vi "Stimulus-Plot (full).vi"(0 "AO Control":T1[](xcontrol), 1 "Waveform Graph":refnum<vi>, 5 "Array":dbl[][](array[numeric]), 9 "Sampling Rate (Hz)":dbl, 11 "error in (no error)":errorcluster, 12 "Decorations[]":refnum<vi>[](array[refnum])) -> (4 "AO Control out":T1[](xcontrol), 6 "Array out":dbl[][](array[numeric]), 15 "error out":errorcluster)   [LabVIEW 2020]
doc: "Helper function to plot stimuli in a sensible fashion."
uses:
  Controls/Multichannel (Full)/Multichannel (Full).xctl
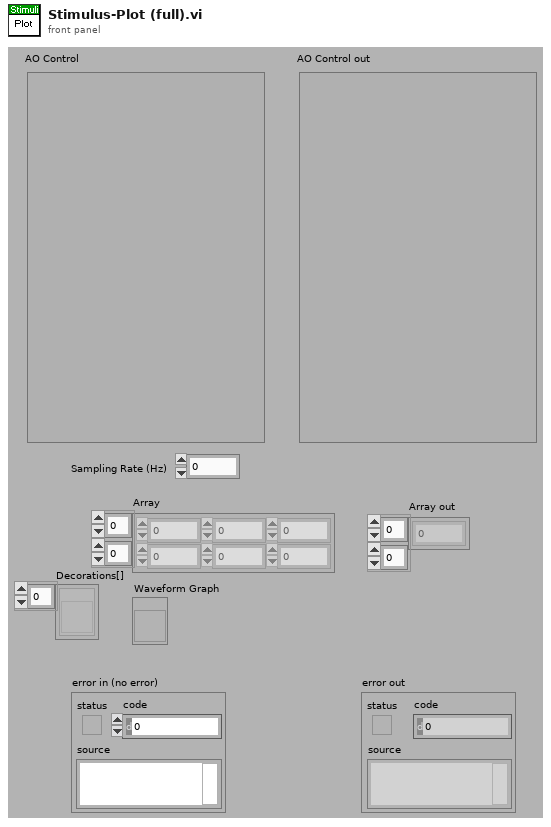
[diagram p1: front panel]
types:
  T1 = typedef "Stimulus Channel (Full).xctl/Full Stimulus Channel Data.ctl" = cluster{"Waveform":T2, "Filter":T19, "Burst":T21, "Level":T22, "Name":string, "Advanced":T24, "SAM":T25}
  T2 = typedef "Waveform XCtl.xctl/Waveform Data.ctl" = cluster{"Type":T3, "Tone":T4, "Pulse Train":T5, "Noise":T8, "File":T9, "FMSweep":T10, "Chirp Train":T11, "Complex Tone":cluster{"Params":T13, "Data":T15}, "Moving Ripple":T16}
  T3 = typedef "Waveform Enum.ctl" = enum16{"OFF", "Tone", "Noise", "Pulse Train", "File", "FM Sweep", "Chirp Train", "Complex Tone", "FM Tone", "Moving Ripple"}
  T4 = typedef "Tone Params.ctl" = cluster{"Frequency (kHz)":dbl, "Last Freq":dbl, "Last Phase":dbl}
  T5 = typedef "Pulse Train Params.ctl" = cluster{"Pulse width (us)":dbl, "Pulse rate (Hz)":dbl, "Gap (ms)":dbl, "Polarity":T6, "PT State":T7, "Asynch":bool}
  T6 = typedef "Pulse Polarity.ctl" = enum16{"POS", "NEG", "POS-NEG", "NEG-POS"}
  T7 = typedef "PT-Continuous State.ctl" = cluster{"Template":dbl[], "Nperiod":i32, "Index":i32, "Pulse Rate (Hz)":dbl, "Phase (cycles)":dbl, "Noff":i32}
  T8 = typedef "Noise Params.ctl" = cluster{"InvFilt":bool, "Noise":dbl[], "CurPt":i32, "Aweight":bool, "Seed":i32, "afile":path}
  T9 = typedef "StimFile-Params.ctl" = cluster{"Filename":path, "Signal":dbl[], "Channel":i32, "stream":bool, "offset":i32, "nreps":i32, "loops":i32, "Randomize":bool, "order":i32[], "Seed":i32, "Tokens":i32}
  T10 = typedef "FM Sweep Params.ctl" = cluster{"Rate (oct/s)":dbl, "Fmin (Hz)":dbl, "Fmax (Hz)":dbl, "Ramp (ms)":dbl, "Linear":bool}
  T11 = typedef "Chirp Train.ctl" = cluster{"Params":T12, "Data":cluster{"WF":dbl[]}}
  T12 = typedef "Chirp Train Params.ctl" = cluster{"Fmin (kHz)":dbl, "Fmax (kHz)":dbl, "Compensate":bool, "Duration (ms)":dbl}
  T13 = typedef "CT-Params.ctl" = cluster{"F0 (Hz)":dbl, "Band":cluster{"Flow (Hz)":dbl, "Fhigh (Hz)":dbl}, "Phase":T14, "Min F0 (Hz)":dbl, "Max F0 (Hz)":dbl, "ContinRandPhase":bool, "Max peak factor":dbl, "Max mod depth":dbl, "MinHarmNum":i32, "MaxHarmNum":i32, "Level Mode":enum16{"per component", "overall rms"}, "% jitter":dbl}
  T14 = typedef "CT-Phase Enum.ctl" = enum16{"Cosine", "Random", "Alternating"}
  T15 = typedef "CT-Runtime Data.ctl" = cluster{"Ncomp":i32, "MinHarm":i32, "Phase":dbl[], "Amplitude":dbl[], "Npts/frame":i32, "Last F0":dbl, "Fmin":dbl, "Fmax":dbl, "Lslope":dbl, "randphase":bool, "overall rms":bool, "fmult":dbl[], "jittered":bool}
  T16 = typedef "Moving Ripple.ctl" = cluster{"Params":T17, "Data":T18}
  T17 = typedef "Moving Ripple.Params.ctl" = cluster{"Fmin":dbl, "Fmax":dbl, "Density":dbl, "Velocity":dbl, "Depth":dbl, "Phase":dbl, "Comp/oct":i32}
  T18 = typedef "Moving Ripple.Data.ctl" = cluster{"Freq":dbl[], "A":dbl[], "phase":dbl[], "Phase":dbl}
  T19 = typedef "Advanced Filter XCtl.xctl/Filter Data.ctl" = cluster{"Type":enum16{"Lowpass", "Highpass", "Bandpass", "Bandstop", "OFF"}, "CF (kHz)":dbl, "BW (kHz)":dbl, "Cascade":bool, "Quadrature":bool, "Scale Factor":dbl, "Stages":cluster{"IIR Filter":cluster{"filter structure":enum32{"IIR 2nd Order", "IIR 4th Order"}, "Reverse Coefficients":dbl[], "Forward Coefficients":dbl[]}, "State":dbl[]}[], "Class":enum16{"Elliptic", "Butterworth"}, "Order":i32, "BWUnits":T20}
  T20 = typedef "Filter-Bandwidth Units.ctl" = enum16{"Linear", "Octaves", "Min-Max"}
  T21 = typedef "Burst Control.xctl/Burst Data.ctl" = cluster{"Active":bool, "Delay (ms)":dbl, "Duration (ms)":dbl, "Ramp (ms)":dbl, "Rate (Hz)":dbl, "Trepeat (ms)":dbl, "Repeat":bool}
  T22 = typedef "Level XCtl.xctl/Level Data.ctl" = cluster{"Level":dbl, "Units":T23, "Max":dbl, "Multiplier":dbl, "Cal File":path, "Cal":cluster{"Freq (Hz)":dbl[], "Mag (dB SPL)":dbl[], "Phase (deg)":dbl[]}}
  T23 = typedef "Level Units.ctl" = enum16{"dB atten", "dB SPL", "dB re 1 Vrms", "dB V/Hz½", "mW", "dB HL", "Volts", "dB mW"}
  T24 = typedef "Advanced Stimulus Options.xctl/Advanced Stimulus Options.ctl" = cluster{"Rep Mask":string, "AltPol":bool, "Var":string, "Expr":string, "Persist":bool}
  T25 = typedef "SAM Params.ctl" = cluster{"Active":bool, "Frequency (Hz)":dbl, "Depth":dbl, "Init Phase (cycles)":dbl, "phase (degrees)":dbl, "Asynch":bool}
  T26 = typedef "LVPoint32TypeDef.ctl" = cluster{"Horizontal":i32, "Vertical":i32}
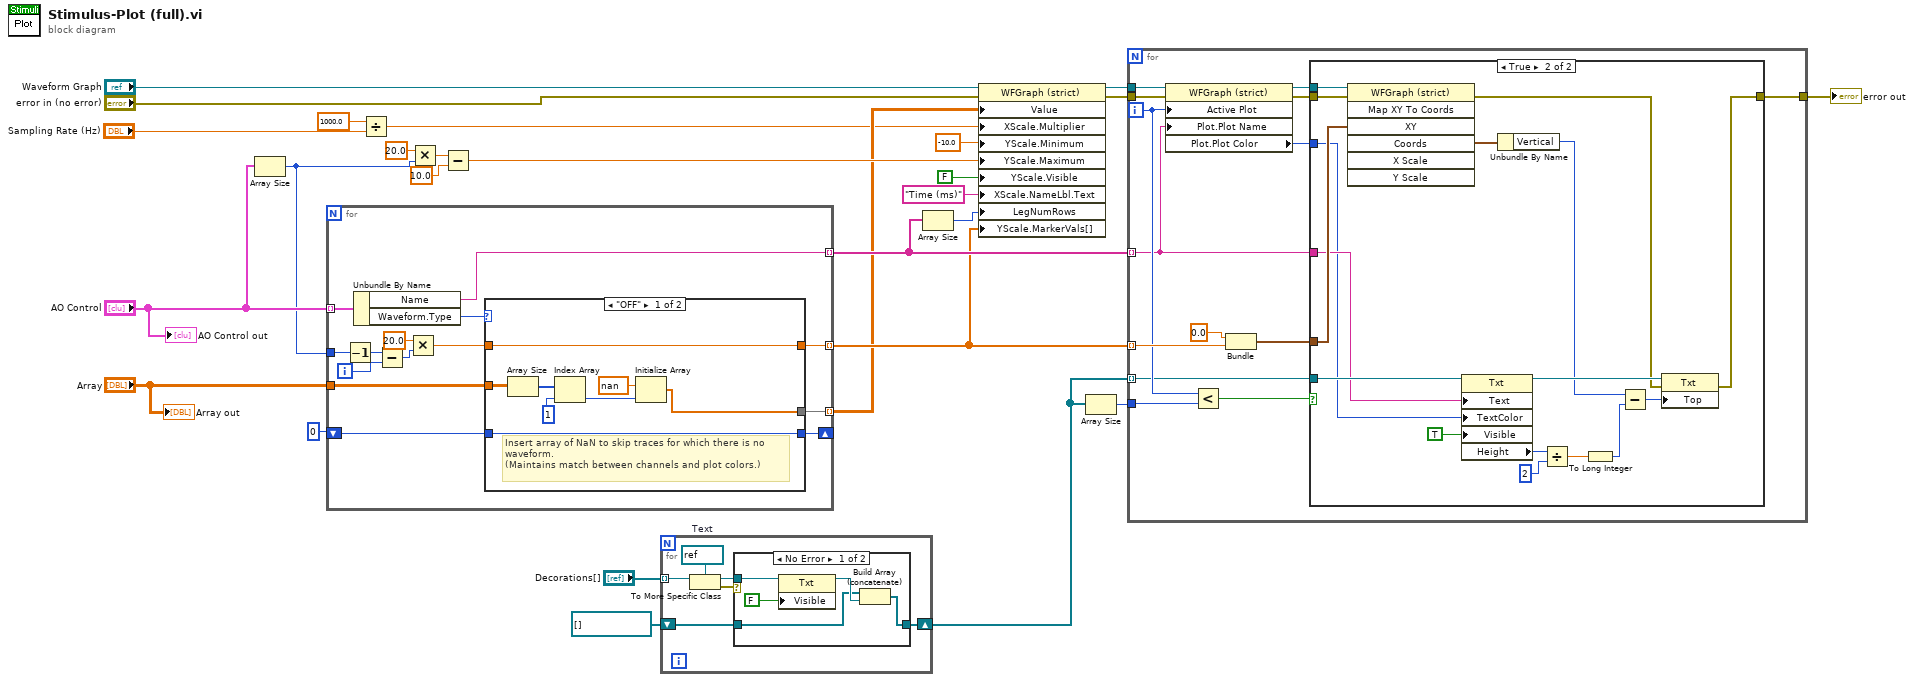
[diagram p0: block diagram]
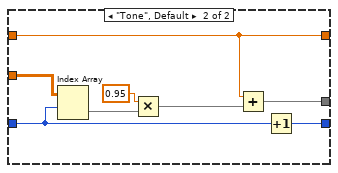
[diagram p4: hidden frame]
diagram:
  n1 = Array Size(array="AO Control") -> (size(s)=w16:i32)
  n2 = for {
    tunnel: "AO Control" -> [w41] mode=indexing
    shift-right: [w38] -> _
    shift-left: 0 -> [w39]
    tunnel: "Array" -> [w37]
    tunnel: [w36] -> w2 mode=indexing
    tunnel: w16 -> [w34]
    tunnel: [w29] -> w9 mode=indexing
    tunnel: [w28] -> w8 mode=indexing
    i -> [w33]
    n3 = Decrement(x=w34) -> (x-1=w30:i32)
    n4 = Unbundle By Name(w41) -> ("Name"=w29:string, "Waveform.Type"=w40:T3)
    n5 = Subtract(x=w30, y=w33) -> (x-y=w32:i32)
    n6 = Multiply(x=20.0, y=w32) -> (x*y=w31:dbl)
    n7 = case shown="\"OFF\"" w40 {
      tunnel: w39 -> [w49 w53]
      tunnel: [w49 w57] -> w38
      tunnel: w37 -> [w48 w55]
      tunnel: [w43 w56] -> w36
      tunnel: w31 -> [w42 w50]
      tunnel: [w42 w50] -> w28
      frame "OFF" {
        # "Insert array of NaN to skip traces for which there is no waveform. \n(Maintains match between channels and plot colors.)"
        n8 = Array Size(array=w48) -> (size(s)=w47:i32[])
        n9 = Index Array(array=w47, index=1) -> (element=w45:i32)
        n10 = Initialize Array(nan ("element"), w45) -> (w43:dbl[])
      }
      frame "Tone", Default {
        n11 = Index Array(array=w55, index (row)=w53) -> (element=w54:dbl[])  [unwired: 1 in]
        n12 = Multiply(x=0.95, y=w54) -> (x*y=w52:dbl[])
        n13 = Add(x=w50, y=w52) -> (x+y=w56:dbl[])
        n14 = Increment(x=w53) -> (x+1=w57:i32)
      }
    }
  }
  n15 = Divide(x=1000.0, y="Sampling Rate (Hz)") -> (x/y=w1:dbl)
  n16 = Multiply(x=20.0, y=w16) -> (x*y=w15:dbl)
  n17 = Subtract(x=w15, y=10.0) -> (x-y=w13:dbl)
  n18 = for {
    tunnel: "Decorations[]" -> [w62] mode=indexing
    shift-right: [w58] -> w6
    shift-left: refnum<vi>[] [] -> [w59]
    w63 = refnum<vi> refnum  # Text
    n19 = To More Specific Class(target class=w63, reference=w62) -> (specific class reference=w61:refnum<vi>, error out=w60:errorcluster)  [unwired: 1 in]
    n20 = case shown="No Error" w60 {
      tunnel: w61 -> [w68 _]
      tunnel: [w64 w69] -> w58
      tunnel: w59 -> [w65 w69]
      frame No Error {
        n21 = property class="Txt"(reference=w68, "Visible"=FALSE) -> (reference out=w66:refnum<vi>)  [unwired: 1 in, 1 out]
        n22 = Build Array (concatenate)(w65, w66) -> (w64:refnum<vi>[])
      }
      frame Error {
      }
    }
  }
  n23 = Array Size(array=w9) -> (size(s)=w11:i32)
  n24 = property class="WFGraph (strict)"(reference="Waveform Graph", error in="error in (no error)", "Value"=w2, "XScale.Multiplier"=w1, "YScale.Minimum"=-10.0 ("Y Scale.Range:Minimum"), "YScale.Maximum"=w13, "YScale.Visible"=FALSE ("Y Scale.Name Label.Visible"), "XScale.NameLbl.Text"="Time (ms)" ("X Scale.Name Label.Text"), "LegNumRows"=w11, "YScale.MarkerVals[]"=w8) -> (reference out=w10:refnum<vi>, error out=w12:errorcluster)
  n25 = Array Size(array=w6) -> (size(s)=w5:i32)
  n26 = for {
    tunnel: w10 -> [w83]
    tunnel: w12 -> [w82]
    tunnel: w9 -> [w73] mode=indexing
    tunnel: w8 -> [w79] mode=indexing
    tunnel: w6 -> [w74] mode=indexing
    tunnel: w5 -> [w76]
    tunnel: [w71] -> w4
    i -> [w77]
    n27 = property class="WFGraph (strict)"(reference=w83, error in=w82, "Active Plot"=w77, "Plot.Plot Name"=w73) -> (reference out=w81:refnum<vi>, error out=w80:errorcluster, "Plot.Plot Color"=w72:u32)
    n28 = Less?(x=w77, y=w76) -> (x < y?=w75:bool)
    n29 = Bundle(0.0, w79) -> (w78:cluster{dbl, dbl})  [unwired: 1 in]
    n30 = case shown="True" w75 {
      tunnel: w81 -> [_ w101]
      tunnel: w80 -> [w84 w100]
      tunnel: w78 -> [_ w99]
      tunnel: w74 -> [_ w98]
      tunnel: w73 -> [_ w97]
      tunnel: w72 -> [_ w95]
      tunnel: [w84 w86] -> w71
      frame False {
      }
      frame True {
        n31 = invoke class="WFGraph (strict)" method="Map XY To Coords"(reference=w101, error in=w100, "XY"=w99) -> (error out=w85:errorcluster, "Coords"=w94:T26)  [unwired: 4 in, 5 out]
        n32 = property class="Txt"(reference=w98, "Text"=w97, "TextColor"=w95, "Visible"=TRUE) -> (reference out=w91:refnum<vi>, "Height"=w93:u32)  [unwired: 1 in, 1 out]
        n33 = Unbundle By Name(w94) -> ("Vertical"=w88:i32)
        n34 = Divide(x=w93, y=u32 2) -> (x/y=w89:dbl)
        n35 = To Long Integer(number=w89) -> (32bit integer=w87:i32)
        n36 = Subtract(x=w88, y=w87) -> (x-y=w90:i32)
        n37 = property class="Txt"(reference=w91, error in=w85, "Top"=w90) -> (error out=w86:errorcluster)  [unwired: 1 out]
      }
    }
  }
  "error out" <- w4
  "AO Control out" <- "AO Control"
  "Array out" <- "Array"
